vi "SUB_OUT_String_token.vi"(3 "input string":string) -> (1 "result string":string)   [LabVIEW 2011]
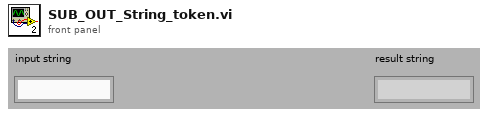
[diagram p1: front panel]
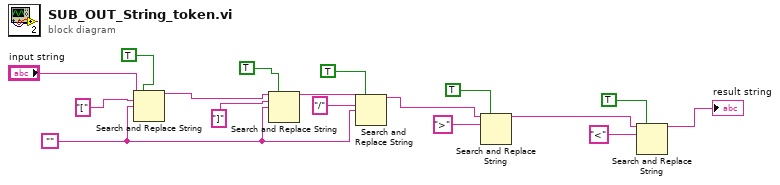
[diagram p0: block diagram]
diagram:
  w9 = ""
  n1 = Search and Replace String(replace all?=TRUE ("replace all? (F)"), input string="input string", search string="[", replace string=w9) -> (result string=w17:string)  [unwired: 4 in, 3 out]
  n2 = Search and Replace String(replace all?=TRUE ("ignore case? (F)"), input string=w17, search string="]", replace string=w9) -> (result string=w11:string)  [unwired: 4 in, 3 out]
  n3 = Search and Replace String(replace all?=TRUE ("replace all? (F)"), input string=w11, search string="/", replace string=w9) -> (result string=w5:string)  [unwired: 4 in, 3 out]
  n4 = Search and Replace String(replace all?=TRUE ("replace all? (F)"), input string=w5, search string=">") -> (result string=w2:string)  [unwired: 5 in, 3 out]
  n5 = Search and Replace String(replace all?=TRUE ("replace all? (F)"), input string=w2, search string="<") -> (result string=→"result string":string)  [unwired: 5 in, 3 out]
